vi "Get Dual Exposure Times.vi"(10 "exposure2":sgl, 11 "exposure1":sgl) -> (1 "function return":u32, 2 "exposure2 out":sgl, 3 "exposure1 out":sgl)   [LabVIEW 2018, in "Copy of Andor SDK.lvlib"]
doc: "EXPNETTYPE unsigned int WINAPI GetDualExposureTimes(float * exposure1, float * exposure2);"
uses:
  Copy of Andor SDK.lvlib
  <userlib>/Andor SDK/ATMCD32D.dll
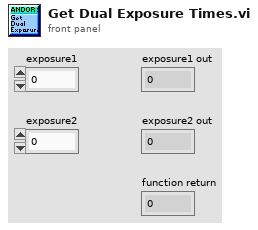
[diagram p1: front panel]
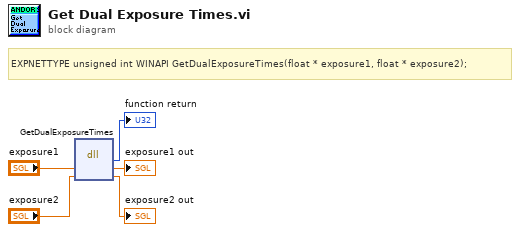
[diagram p0: block diagram]
diagram:
  # "EXPNETTYPE unsigned int WINAPI GetDualExposureTimes(float * exposure1, float * exposure2);"
  n1 = dll-call lib="C:/Program Files (x86)/National Instruments/LabVIEW 2018/user.lib/Andor SDK/ATMCD32D.*" fn="GetDualExposureTimes"("exposure1"="exposure1", "exposure2"="exposure2") -> (→"function return":u32, "exposure1"=→"exposure1 out":sgl, "exposure2"=→"exposure2 out":sgl)  [unwired: 3 in, 2 out]
